vi "Voltage and Current Ring Chooser.vi"(8 "error in (no error)":errorcluster, 11 "Generic Instrument in":refnum<class "Generic Instrument.lvclass">) -> (0 "error out":errorcluster, 3 "Generic Instrument out":refnum<class "Generic Instrument.lvclass">)   [LabVIEW 2014, in "Generic Instrument.lvlib" / "Generic Instrument.lvclass"]
uses:
  Generic Instrument.lvclass
  <vilib>/Utility/miscctls.llb/LVStringsAndValuesArrayTypeDef_U16.ctl
panel:
  out "Wiring Strings And Values []":T1
  in  "Wiring":u16(ring)
  out "Current Strings And Values []":T1
  out "Voltage Strings And Values []":T1
  in  "Current":u16(ring)
  in  "Voltage":u16(ring)
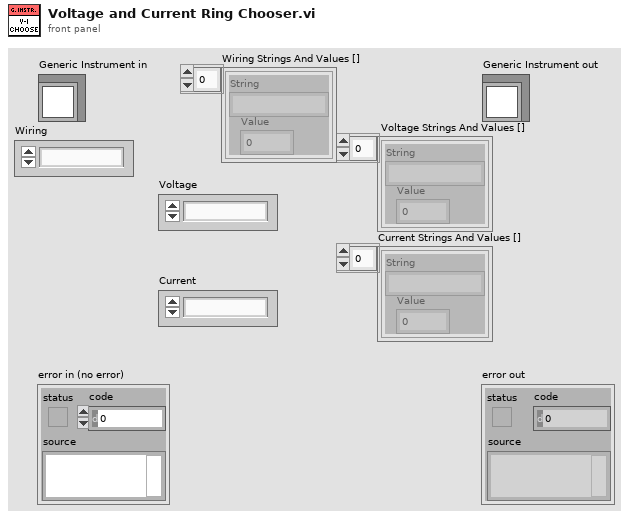
[diagram p1: front panel]
types:
  T1 = typedef "LVStringsAndValuesArrayTypeDef_U16.ctl" = cluster{"String":string, "Value":u16}[]
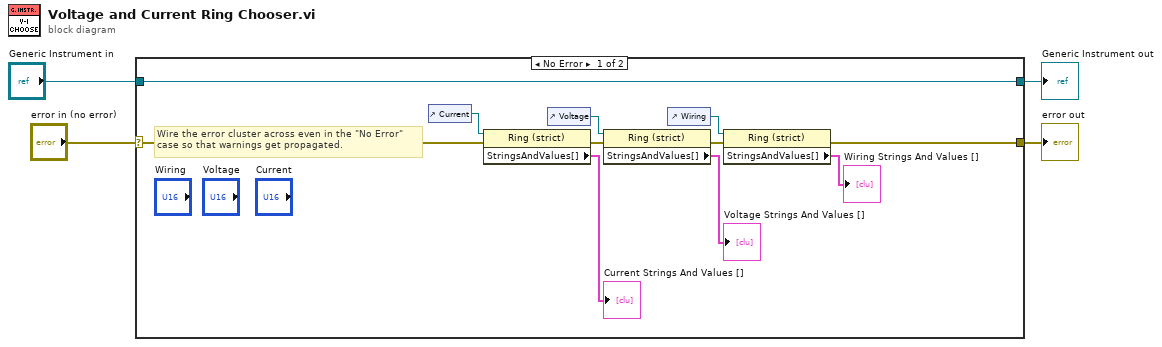
[diagram p0: block diagram]
diagram:
  n1 = case shown="No Error" "error in (no error)" {
    selector: "error in (no error)" -> [w10 w17]
    tunnel: [w7 w17] -> w3
    tunnel: [w15 w16] -> w1
    tunnel: "Generic Instrument in" -> [w15 w16]
    frame No Error {
      # "Wire the error cluster across even in the \"No Error\"\ncase so that warnings get propagated."
      n2 = control-ref of="Current"() -> (w12:refnum<vi>)
      n3 = property class="Ring (strict)"(reference=w12, error in=w10) -> (error out=w11:errorcluster, "StringsAndValues[]"=→"Current Strings And Values []":T1)  [unwired: 1 out]
      n4 = control-ref of="Voltage"() -> (w14:refnum<vi>)
      n5 = property class="Ring (strict)"(reference=w14, error in=w11) -> (error out=w8:errorcluster, "StringsAndValues[]"=→"Voltage Strings And Values []":T1)  [unwired: 1 out]
      n6 = control-ref of="Wiring"() -> (w6:refnum<vi>)
      n7 = property class="Ring (strict)"(reference=w6, error in=w8) -> (error out=w7:errorcluster, "StringsAndValues[]"=→"Wiring Strings And Values []":T1)  [unwired: 1 out]
    }
    frame Error {
    }
  }
  "error out" <- w3
  "Generic Instrument out" <- w1
